vi "PDC Configure Hardware.vi"(0 "VISA Resource Name":refnum<visa-resource-name>, 5 "Optimize RNYQ For (T:EVM)":bool=TRUE, 7 "EXT Data Clock (T:NORMAL)":bool=TRUE, 9 "BBG Data Clock (F:INT)":bool, 11 "error in (no error)":errorcluster {"code" format="%.0x"}) -> (4 "VISA Resource Name Out":refnum<visa-resource-name>, 15 "error out":errorcluster {"code" format="%.0x"})   [LabVIEW 2012, in "Agilent ESG Series.lvlib"]
doc: "This VI is used to configure the \"Configure Hardware\" parameters."
uses:
  <instrlib>/Agilent ESG Series/Agilent ESG Series.lvlib
panel:
  # "EVM"
  # "ACP"
  # "NORMAL"
  # "SYMBOL"
  # "EXT"
  # "INT"
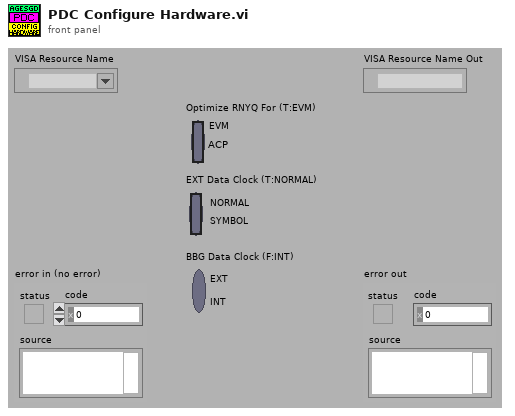
[diagram p1: front panel]
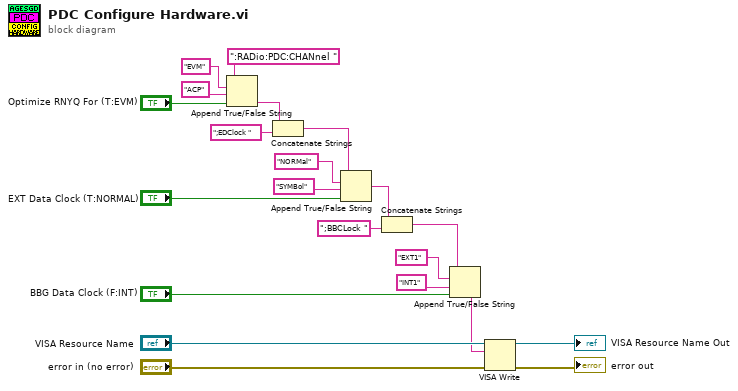
[diagram p0: block diagram]
diagram:
  n1 = Append True/False String(1:"Optimize RNYQ For (T:EVM)", 2:"ACP" ("false string"), 3:"EVM" ("true string"), 4:":RADio:PDC:CHANnel ") -> (0:w10:string)
  n2 = Concatenate Strings(w10, ";EDClock ") -> (w11:string)
  n3 = Append True/False String(1:"EXT Data Clock (T:NORMAL)", 2:"SYMBol" ("false string"), 3:"NORMal" ("true string"), 4:w11) -> (0:w4:string)
  n4 = Concatenate Strings(w4, ";BBCLock ") -> (w5:string)
  n5 = Append True/False String(1:"BBG Data Clock (F:INT)", 2:"INT1" ("false string"), 3:"EXT1" ("true string"), 4:w5) -> (0:w2:string)
  n6 = VISA Write(VISA resource name="VISA Resource Name", write buffer=w2, error in (no error)="error in (no error)") -> (VISA resource name out=→"VISA Resource Name Out":refnum<visa-resource-name>, error out=→"error out":errorcluster)  [unwired: 1 out]
